vi "TSPopup.Lookup.vi"(8 "error in (no error)":errorcluster, 9 "Point":cluster{"X":i32, "Y":i32}, 11 "Ctl Refnum":refnum<vi>) -> (0 "error out":errorcluster, 1 "In Bounds?":bool, 2 "Found":bool, 3 "Popup Parameters":T3, 4 "Cell Info (Call data)":T1)   [LabVIEW 2013]
doc: "Searches the registered controls for Popup Parameters (type) associated with the location that was clicked on. Search order is : Exact Cell, Entire Column, Entire Row, Entire Control.\n\n<B>Ctl Refnum</B> - Refnum of the control that was clicked on. This same reference should have been used to register parameters using \"TSPopup.Register.vi\"\n<B>Point</B> - Mouse coordinates of <B>Mouse Down?</B> Event.\n\n<B>Popup Parameters</B> - Parameters for showing the Type Sensitive Popup.\n<B>Found</B> - Indicates whether the clicked location had parameters registered.\n<B>In Bounds?</B> - Indicates whether the mouse click was within main area of control (not the label, caption, scrollbars, etc.).\n<B>Cell Info (Call data)</B> - This provides helpful information for editing the Popup Parameters and for sending as the Call Data.\n\nType Sensitive Popup \nCopyright © 2007, J. David Saunders\nAll rights reserved."
uses:
  TSPopup.Popup Call Parameters.ctl
  TSPopup.Data Type.ctl
  TSPopup.Grid.Cell Info.ctl
  Private/TSPopup.Popup Operation.ctl
panel:
  # "Type Sensitive Popup \nCopyright © 2007, J. David Saunders\nAll rights reserved."
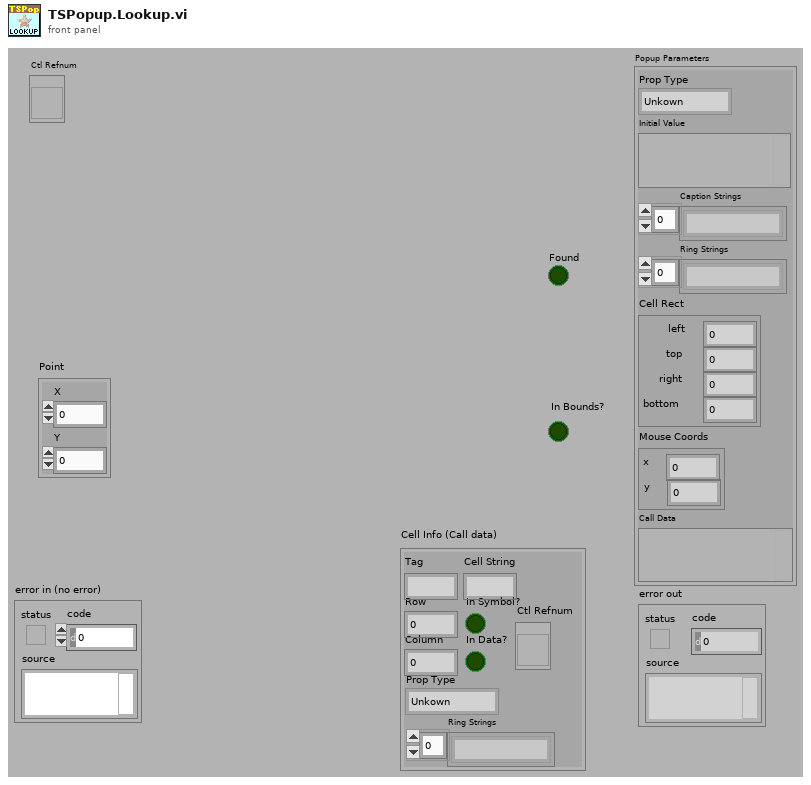
[diagram p1: front panel]
types:
  T1 = typedef "TSPopup.Grid.Cell Info.ctl" = cluster{"Tag":string, "Row":i32, "Column":i32, "In Symbol?":bool, "In Data?":bool, "Cell String":string, "Ctl Refnum":refnum<vi>, "Prop Type":T2, "Ring Strings":string[]}
  T2 = typedef "TSPopup.Data Type.ctl" = enum16{"Unkown", "NO POPUP", "String", "Integer", "Float", "Color", "Boolean", "Ring", "Captioned String", "Captioned Integer", "Button Color", "2 Int Cluster", "4 Int Cluster"}
  T3 = typedef "TSPopup.Popup Call Parameters.ctl" = cluster{"Prop Type":T2, "Initial Value":variant, "Caption Strings":string[], "Ring Strings":string[], "Cell Rect":cluster{"left":i16, "top":i16, "right":i16, "bottom":i16}, "Mouse Coords":cluster{"x":i16, "y":i16}, "Call Data":variant}
  T4 = typedef "TSPopup.Popup Operation.ctl" = enum16{"Show", "Initialize", "Close", "Popup Done", "Register a Location's Type", "Retrieve Location's Type"}
  T5 = cluster{"left":i16, "top":i16, "right":i16, "bottom":i16}
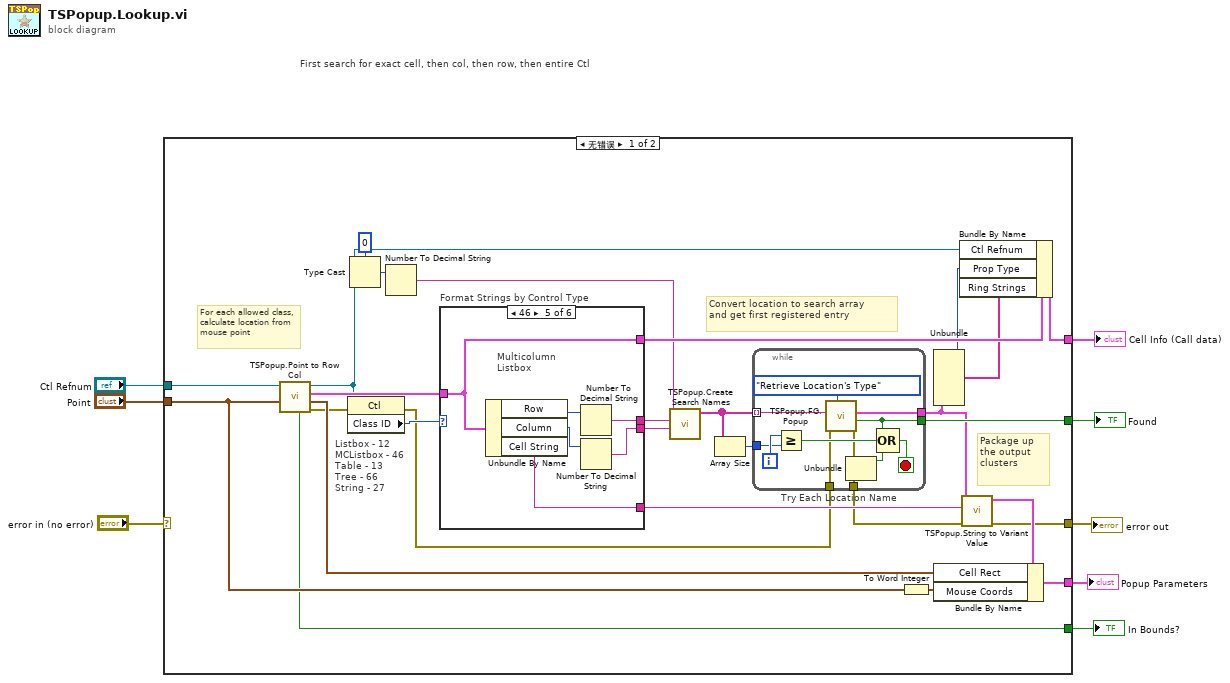
[diagram p0: block diagram]
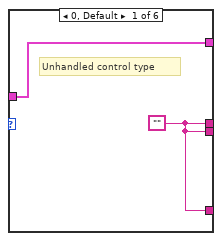
[diagram p2: hidden frame]
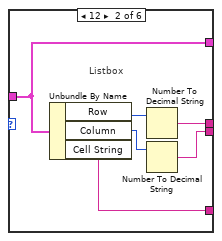
[diagram p3: hidden frame]
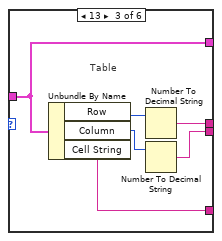
[diagram p4: hidden frame]
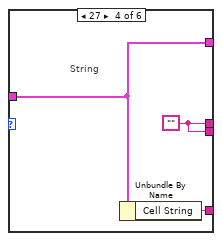
[diagram p5: hidden frame]
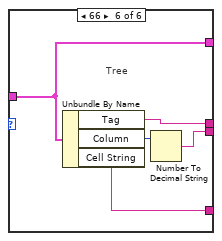
[diagram p6: hidden frame]
diagram:
  # "First search for exact cell, then col, then row, then entire Ctl"
  n1 = case shown="无错误" "error in (no error)" {
    selector: "error in (no error)" -> [_ w76]
    tunnel: [w18 w76] -> w6
    tunnel: "Ctl Refnum" -> [w17 _]
    tunnel: "Point" -> [w15 _]
    tunnel: [w31 _] -> w7
    tunnel: [w26 _] -> w5
    tunnel: [w12 _] -> w4
    tunnel: [w24 _] -> w8
    frame No Error {
      # "Package up\nthe output\nclusters"
      # "Convert location to search array\nand get first registered entry"
      # "For each allowed class,\ncalculate location from\nmouse point"
      # "Listbox - 12\nMCListbox - 46\nTable - 13\nTree - 66\nString - 27"
      n2 = call "TSPopup.Point to Row Col.vi"("Point"=w15, "Grid Ctl Reference In"=w17) -> ("error out"=w11:errorcluster, "Cell Rect Out"=w14:T5, "Cell Info Out"=w16:T1, "Grid Ctl Reference Out"=w9:refnum<vi>, "In Bounds?"=w12:bool)  [unwired: 5 in]
      n3 = property class="Ctl"(reference=w9, error in=w11) -> (error out=w10:errorcluster, "Class ID"=w36:u32)  [unwired: 1 out]
      n4 = Type Cast(type=0, x=w9) -> (*(type *) &x=w34:i32)
      n5 = Number To Decimal String(number=w34) -> (decimal integer string=w13:string)  [unwired: 1 in]
      n6 = case "Format Strings by Control Type" shown="46" w36 {
        tunnel: [w49 w54 w60 w64 w69 w75] -> w30
        tunnel: [w49 w52 w59 w64 w68 w73] -> w29
        tunnel: [w49 w51 w61 w63 w70 w72] -> w25
        tunnel: [w48 w50 w56 w62 w65 w71] -> w23
        tunnel: w16 -> [w48 w50 w56 w62 w65 w71]
        frame 0, Default {
          w49 = ""
          # "Unhandled control type"
        }
        frame 12 {
          # "Listbox"
          n7 = Unbundle By Name(w50) -> ("Row"=w55:i32, "Column"=w53:i32, "Cell String"=w51:string)
          n8 = Number To Decimal String(number=w55) -> (decimal integer string=w54:string)  [unwired: 1 in]
          n9 = Number To Decimal String(number=w53) -> (decimal integer string=w52:string)  [unwired: 1 in]
        }
        frame 13 {
          # "Table"
          n10 = Unbundle By Name(w56) -> ("Row"=w58:i32, "Column"=w57:i32, "Cell String"=w61:string)
          n11 = Number To Decimal String(number=w58) -> (decimal integer string=w60:string)  [unwired: 1 in]
          n12 = Number To Decimal String(number=w57) -> (decimal integer string=w59:string)  [unwired: 1 in]
        }
        frame 27 {
          w64 = ""
          # "String"
          n13 = Unbundle By Name(w62) -> ("Cell String"=w63:string)
        }
        frame 46 {
          # "Multicolumn\nListbox"
          n14 = Unbundle By Name(w65) -> ("Row"=w67:i32, "Column"=w66:i32, "Cell String"=w70:string)
          n15 = Number To Decimal String(number=w67) -> (decimal integer string=w69:string)  [unwired: 1 in]
          n16 = Number To Decimal String(number=w66) -> (decimal integer string=w68:string)  [unwired: 1 in]
        }
        frame 66 {
          # "Tree"
          n17 = Unbundle By Name(w71) -> ("Tag"=w75:string, "Column"=w74:i32, "Cell String"=w72:string)
          n18 = Number To Decimal String(number=w74) -> (decimal integer string=w73:string)  [unwired: 1 in]
        }
      }
      n19 = call "TSPopup.Create Search Names.vi"("Column String"=w29, "Tag or Row String"=w30, "Control Ref String"=w13) -> ("Search Names"=w33:string[])  [unwired: 8 in]
      n20 = Array Size(array=w33) -> (size(s)=w32:i32)
      n21 = while "Try Each Location Name" {
        tunnel: [w47] -> w22
        tunnel: w33 -> [w45] mode=indexing
        tunnel: w32 -> [w43]
        tunnel: [w41] -> w31
        tunnel: w10 -> [w38]
        tunnel: [w37] -> w19
        i -> [w44]
        stop <- w39 stop-if-true
        n22 = Greater Or Equal?(x=w44, y=w43) -> (x >= y?=w42:bool)
        n23 = call "TSPopup.FG.Popup.vi"("Popup Operation"=TSPopup.Popup_Operation."Retrieve Location's Type", "error in (no error)"=w38, "Encoded Location"=w45) -> ("error out"=w37:errorcluster, "Found"=w41:bool, "Popup Parameters out"=w47:T3)  [unwired: 5 in, 1 out]
        n24 = Unbundle(w37) -> ("status"=w40:bool)  [unwired: 2 out]
        n25 = Compound Arithmetic op=OR(w41, w42, w40) -> (w39:bool)
      }
      n26 = To Word Integer(number=w15) -> (16bit integer=w28:cluster{"X":i16, "Y":i16})
      n27 = Unbundle(w22) -> ("Prop Type"=w20:T2, "Ring Strings"=w21:string[])  [unwired: 5 out]
      n28 = Bundle By Name(cluster=w23, "Ctl Refnum"=w9, "Prop Type"=w20, "Ring Strings"=w21) -> (w24:T1)
      n29 = call "TSPopup.String to Variant Value.vi"("error in (no error)"=w19, "Cell String"=w25, "Popup Parameters"=w22) -> ("error out"=w18:errorcluster, "Popup Parameters out"=w27:T3)  [unwired: 6 in, 1 out]
      n30 = Bundle By Name(cluster=w27, "Cell Rect"=w14, "Mouse Coords"=w28) -> (w26:T3)
    }
    frame Error {
    }
  }
  "error out" <- w6
  "Found" <- w7
  "In Bounds?" <- w4
  "Popup Parameters" <- w5
  "Cell Info (Call data)" <- w8
